vi "LVClass_WavefrontCorrectorSet Get Parameter String List One Element.vi"(0 "WavefrontCorrectorSet in":refnum<class "WavefrontCorrectorSet.lvclass">, 5 "parameter name":string, 7 "index":u32, 11 "error in (no error)":errorcluster) -> (4 "WavefrontCorrectorSet out":refnum<class "WavefrontCorrectorSet.lvclass">, 6 "value":string, 15 "error out":errorcluster)   [LabVIEW 2020, in "WavefrontCorrectorSet.lvclass"]
doc: "If parameter is a string to be selected among a finite set of strings,\nextract the possible value located at the /p index position from this set.\nSee Imop_WavefrontCorrectorSet_GetParameterOption.\n\n--------------------------------------------------------------------------------\n\n<B>wavefrontcorrector_setIn </B> : WavefrontCorrectorSet object.\n<B>wavefrontcorrector_setOut </B> : WavefrontCorrectorSet object.\n<B>parameter_name </B> : Parameter name (must be the name of a parameter of type strings list).\n<B>index </B> : Sub-parameter index.\n<B>value </B> : Value at index index.\n<B>ErrorIn </B> : Error\n<B>ErrorOut </B> : Error\n\n--------------------------------------------------------------------------------"
uses:
  WavefrontCorrectorSet.lvclass
  WavefrontCorrectorSet.lvclass/WavefrontCorrectorSet.ctl
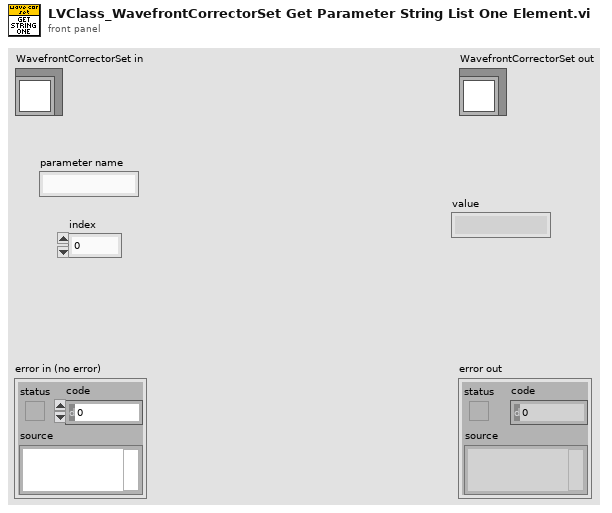
[diagram p1: front panel]
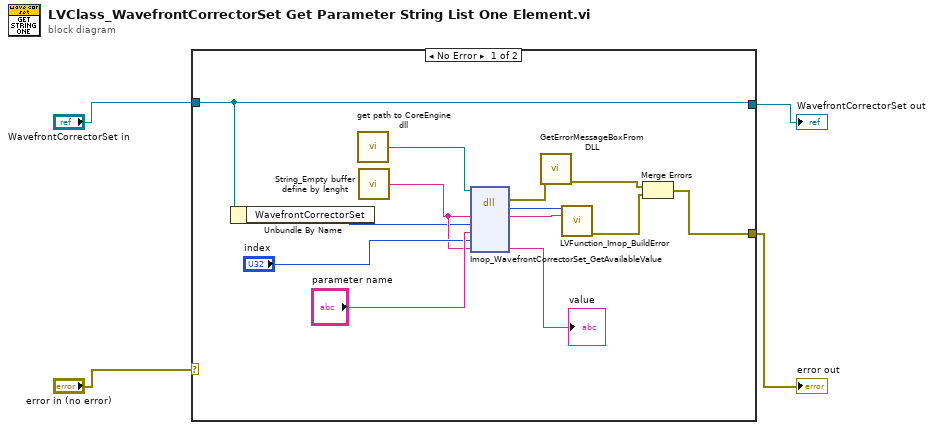
[diagram p0: block diagram]
diagram:
  n1 = case shown="No Error" "error in (no error)" {
    selector: "error in (no error)" -> [_ w18]
    tunnel: "WavefrontCorrectorSet in" -> [w9 w19]
    tunnel: [w9 w19] -> w1
    tunnel: [w5 w18] -> w2
    frame No Error {
      n2 = Unbundle By Name(w9) -> ("WavefrontCorrectorSet"=w8:i32)
      n3 = call "get path to CoreEngine dll.vi"() -> ("path to c_interface_vc100.dll"=w14:path)  [unwired: 12 in, 3 out]
      n4 = call "String_Empty buffer define by lenght.vi"() -> ("Empty buffer"=w11:string)  [unwired: 1 in]
      n5 = dll-call lib="D:/soft/HASO_v3/SVN_trunk/ImOpCoreEngine4_LV2011/DLLs/c_interface_vc100.dll" fn="Imop_WavefrontCorrectorSet_GetAvailableValue"(path in=w14, "message"=w11, "objet"=w8, "parameter name"="parameter name", "index"="index", "Name"=w11) -> (error out=w13:errorcluster, "return type"=w17:i32, "message"=w16:string, "Name"=→"value":string)  [unwired: 5 in, 1 out]
      n6 = call "GetErrorMessageBoxFromDLL.vi"("error IN"=w13) -> ("error OUT"=w7:errorcluster)  [unwired: 10 in]
      n7 = call "LVFunction_Imop_BuildError.vi"("code"=w17, "String to Prepend to source (\"\")"=w16) -> ("error out"=w6:errorcluster)  [unwired: 13 in]
      n8 = Merge Errors(w7, w6) -> (w5:errorcluster)
    }
    frame Error {
    }
  }
  "error out" <- w2
  "WavefrontCorrectorSet out" <- w1
